vi "Position as function of time (SubVI).vi"(9 "v":dbl, 10 "a":dbl, 11 "F(t)":dbl) -> (3 "x(t)":dbl)   [LabVIEW 2024]
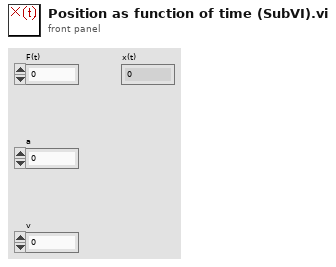
[diagram p1: front panel]
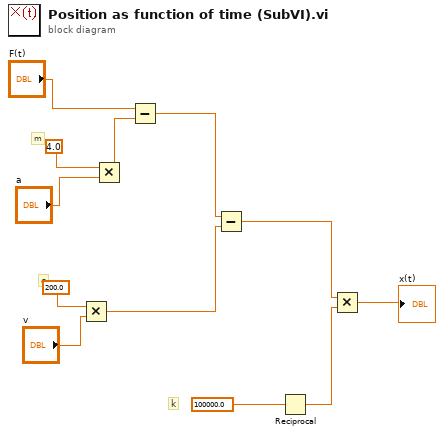
[diagram p0: block diagram]
diagram:
  # "m"
  # "c"
  # "k"
  n1 = Multiply(x=200.0 ("c"), y="v") -> (x*y=w8:dbl)
  n2 = Multiply(x=4.0 ("m"), y="a") -> (x*y=w5:dbl)
  n3 = Subtract(x="F(t)", y=w5) -> (x-y=w9:dbl)
  n4 = Subtract(x=w9, y=w8) -> (x-y=w10:dbl)
  n5 = Reciprocal(x=100000.0 ("k")) -> (1/x=w11:dbl)
  n6 = Multiply(x=w10, y=w11) -> (x*y=→"x(t)":dbl)
